vi "svx_Configure (DAQmx).vi"(0 "acquisition task in":T1={"AI device settings"={"AI DAQmx TaskID"="", "response"=[]}, "acquisition type"=enum."Finite", "measurement settings"={"AI sampling frequency"=0.0, "AO sampling frequency"=0.0, "AI block size"=0, "AO block Size"=0, "block duration [ms]"=100.0, "number of AI channels"=0, "device propagation delay [samples]"=0.0, "DUT propagation time [s]"=0.0}, "settling settings"={"settle time"=0.015599999576807022, "settle cycles"=5}, "integration settings"={"integration time"=0.015599999576807022, "integration cycles"=5}, "AO device settings"={"AO DAQmx taskID"="", "excitation"=[]}, "acquisition accounting"={"initial read size [samples]"=0, "read offset [samples]"=0, "read length [samples]"=0, "blocks to settle [samples]"=0, "min delay until transition [samples]"=0}, "frequency range"={"start frequency"=0.0, "stop frequency"=0.0}, "block type"=enum."Initialize", "source settings"={"signal type"=enum."Sine wave", "frequency"=0.0, "total amplitude"=0.0, "frequencies"=[1.0], "relative amplitudes"=[1.0], "offset"=1.0, "total amplitude list"=[1.0], "ramping rate"=0.0}, "chirp settings"={"amplitude"=1.0, "frequency range"={"start (Hz)"=20.0, "stop (Hz)"=20000.0, "frequency spacing"=enum."Logarithmic"}, "sampling info"={"Fs"=50000.0, "chirp duration [s]"=3.0}, "initial states"={"frequency [Hz]"=20.0, "phase [rad]"=0.0, "elapsed time [s]"=0.0}, "frequency slope"=0.0, "maximum harmonic"=3, "prefix len [samples]"={"integer"=0, "fractional"=0.0}}} {"chirp settings"."frequency slope" format="%.2f"; "chirp settings"."prefix len [samples]"."fractional" format="%.2p"; "chirp settings"."initial states"."elapsed time [s]" format="%.2f"; "chirp settings"."initial states"."phase [rad]" format="%.2f"; "chirp settings"."initial states"."frequency [Hz]" format="%.2f"; "chirp settings"."sampling info"."chirp duration [s]" format="%.2f"; "chirp settings"."sampling info"."Fs" format="%.2p"; "chirp settings"."frequency range"."stop (Hz)" format="%.2f"; "chirp settings"."frequency range"."start (Hz)" format="%.2f"; "chirp settings"."amplitude" format="%.2f"; "source settings"."total amplitude" format="%.2f"; "source settings"."relative amplitudes" format="%.2f"; "source settings"."frequencies" format="%.2f"; "source settings"."total amplitude list" format="%.2f"; "source settings"."ramping rate" format="%.4f"; "source settings"."offset" format="%.2f"; "source settings"."frequency" format="%.2f"; "frequency range"."stop frequency" format="%.2f"; "frequency range"."start frequency" format="%.2f"; "AO device settings"."excitation"."AO channel settings"."terminal config" items=["Default"=-1, "Differential"=10106, "Pseudodifferential"=12529]; "AI device settings"."response"."AI channel settings"."DSA channel settings"."IEPE current [mA]" min=0.0 max=20.0 format="%.1f"; "AI device settings"."response"."AI channel settings"."DSA channel settings"."coupling" items=["AC"=10045, "DC"=10050, "GND"=10066]; "AI device settings"."response"."AI channel settings"."min value [V]" format="%.2f"; "AI device settings"."response"."AI channel settings"."terminal config" items=["Default"=-1, "RSE"=10083, "NRSE"=10078, "Differential"=10106, "Pseudodifferential"=12529]; "AI device settings"."response"."AI channel settings"."max value [V]" format="%.2f"; "integration settings"."integration time" format="%.2p"; "settling settings"."settle time" format="%.2p"; "measurement settings"."DUT propagation time [s]" format="%.2f"; "measurement settings"."AO sampling frequency" format="%.2f"; "measurement settings"."AI sampling frequency" format="%.2f"}, 11 "error in (no error)":errorcluster) -> (4 "acquisition task out":T1={"AI device settings"={"AI DAQmx TaskID"="", "response"=[]}, "acquisition type"=enum."Finite", "measurement settings"={"AI sampling frequency"=51200.0, "AO sampling frequency"=51200.0, "AI block size"=0, "AO block Size"=0, "block duration [ms]"=100.0, "number of AI channels"=0, "device propagation delay [samples]"=0.0, "DUT propagation time [s]"=0.0}, "settling settings"={"settle time"=0.015599999576807022, "settle cycles"=5}, "integration settings"={"integration time"=0.015599999576807022, "integration cycles"=5}, "AO device settings"={"AO DAQmx taskID"="", "excitation"=[]}, "acquisition accounting"={"initial read size [samples]"=0, "read offset [samples]"=0, "read length [samples]"=0, "blocks to settle [samples]"=0, "min delay until transition [samples]"=0}, "frequency range"={"start frequency"=0.015599999576807022, "stop frequency"=5.0}, "block type"=enum."Initialize", "source settings"={"signal type"=enum."Sine wave", "frequency"=5.0, "total amplitude"=0.0, "frequencies"=[1.0], "relative amplitudes"=[1.0], "offset"=1.0, "total amplitude list"=[1.0], "ramping rate"=0.0}, "chirp settings"={"amplitude"=1.0, "frequency range"={"start (Hz)"=20.0, "stop (Hz)"=20000.0, "frequency spacing"=enum."Logarithmic"}, "sampling info"={"Fs"=50000.0, "chirp duration [s]"=3.0}, "initial states"={"frequency [Hz]"=20.0, "phase [rad]"=0.0, "elapsed time [s]"=0.0}, "frequency slope"=0.0, "maximum harmonic"=3, "prefix len [samples]"={"integer"=0, "fractional"=0.0}}} {"chirp settings"."frequency slope" format="%.2f"; "chirp settings"."prefix len [samples]"."fractional" format="%.2p"; "chirp settings"."initial states"."elapsed time [s]" format="%.2f"; "chirp settings"."initial states"."phase [rad]" format="%.2f"; "chirp settings"."initial states"."frequency [Hz]" format="%.2f"; "chirp settings"."sampling info"."chirp duration [s]" format="%.2f"; "chirp settings"."sampling info"."Fs" format="%.2p"; "chirp settings"."frequency range"."stop (Hz)" format="%.2f"; "chirp settings"."frequency range"."start (Hz)" format="%.2f"; "chirp settings"."amplitude" format="%.2f"; "source settings"."total amplitude" format="%.2f"; "source settings"."relative amplitudes" format="%.2f"; "source settings"."frequencies" format="%.2f"; "source settings"."total amplitude list" format="%.2f"; "source settings"."ramping rate" format="%.4f"; "source settings"."offset" format="%.2f"; "source settings"."frequency" format="%.2f"; "frequency range"."stop frequency" format="%.2f"; "frequency range"."start frequency" format="%.2f"; "AO device settings"."excitation"."AO channel settings"."terminal config" items=["Default"=-1, "Differential"=10106, "Pseudodifferential"=12529]; "AI device settings"."response"."AI channel settings"."DSA channel settings"."IEPE current [mA]" min=0.0 max=20.0 format="%.1f"; "AI device settings"."response"."AI channel settings"."DSA channel settings"."coupling" items=["AC"=10045, "DC"=10050, "GND"=10066]; "AI device settings"."response"."AI channel settings"."min value [V]" format="%.2f"; "AI device settings"."response"."AI channel settings"."terminal config" items=["Default"=-1, "RSE"=10083, "NRSE"=10078, "Differential"=10106, "Pseudodifferential"=12529]; "AI device settings"."response"."AI channel settings"."max value [V]" format="%.2f"; "integration settings"."integration time" format="%.2p"; "settling settings"."settle time" format="%.2p"; "measurement settings"."DUT propagation time [s]" format="%.2f"; "measurement settings"."AO sampling frequency" format="%.2f"; "measurement settings"."AI sampling frequency" format="%.2f"}, 6 "actual scan rate":dbl format="%.2f", 15 "error out":errorcluster)   [LabVIEW 2017]
uses:
  <vilib>/addons/Sound and Vibration/Example Support/Audio/DAQmx/svx_Acquisition Task (DAQmx).ctl
  <vilib>/addons/_NISVFA/_Shared subVIs/Controls/svc_Channel Settings.ctl
  <vilib>/addons/_NISVFA/_Shared subVIs/Controls/svc_DSA Channel Settings.ctl
  <vilib>/addons/_NISVFA/_Generation/subVIs/sv_Chirp Settings.ctl
  <vilib>/DAQmx/configure/trigger.llb/DAQmx Start Trigger (Digital Edge).vi
  <vilib>/DAQmx/configure/timing.llb/DAQmx Timing (Sample Clock).vi
  <vilib>/DAQmx/create/channels.llb/DAQmx Create Channel (AO-Voltage-Basic).vi
  <vilib>/DAQmx/create/channels.llb/DAQmx Create Channel (AI-Voltage-Basic).vi
  <resource>/objmgr/daqmx.rc
  <vilib>/addons/_NISVFA/_Generation/SoundVib_Generation.lvlib
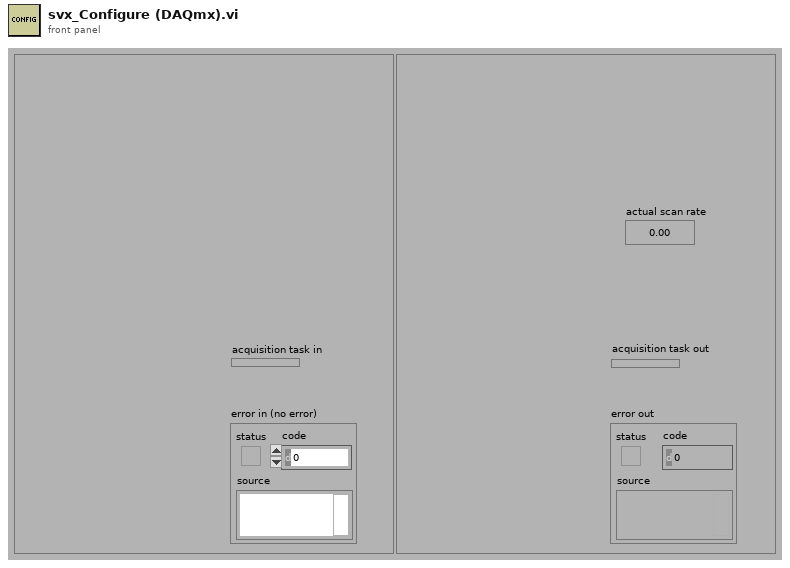
[diagram p1: front panel]
types:
  T1 = typedef "svx_Acquisition Task (DAQmx).ctl" = cluster{"AI device settings":cluster{"AI DAQmx TaskID":refnum<k21>, "response":cluster{"AI physical channel":tag, "AI channel settings":T2}[]}, "acquisition type":enum16{"Finite", "Averaged", "Settled", "Amplitude Sweep", "Stepped Frequency Sweep", "Continuous Frequency Sweep"}, "measurement settings":cluster{"AI sampling frequency":dbl, "AO sampling frequency":dbl, "AI block size":i32, "AO block Size":i32, "block duration [ms]":dbl, "number of AI channels":i32, "device propagation delay [samples]":dbl, "DUT propagation time [s]":dbl}, "settling settings":cluster{"settle time":dbl, "settle cycles":i32}, "integration settings":cluster{"integration time":dbl, "integration cycles":i32}, "AO device settings":cluster{"AO DAQmx taskID":refnum<k21>, "excitation":cluster{"AO physical channel":tag, "AO channel settings":cluster{"maximum value (10 V)":dbl, "minimum value (10 V)":dbl, "terminal config":i32}}[]}, "acquisition accounting":cluster{"initial read size [samples]":i32, "read offset [samples]":i32, "read length [samples]":i32, "blocks to settle [samples]":i32, "min delay until transition [samples]":i32}, "frequency range":cluster{"start frequency":dbl, "stop frequency":dbl}, "block type":enum16{"Initialize", "Settle", "Integrate"}, "source settings":cluster{"signal type":enum16{"Sine wave", "Dual tone (IMD)", "Multitone", "Chirp", "Frequency flat chirp", "Uniform white noise", "Gaussian white noise", "Pink noise", "PRN", "Continuous swept-sine"}, "frequency":dbl, "total amplitude":dbl, "frequencies":dbl[], "relative amplitudes":dbl[], "offset":dbl, "total amplitude list":dbl[], "ramping rate":dbl}, "chirp settings":T4}
  T2 = typedef "svc_Channel Settings.ctl" = cluster{"max value [V]":dbl, "min value [V]":dbl, "terminal config":i32, "DSA channel settings":T3}
  T3 = typedef "svc_DSA Channel Settings.ctl" = cluster{"coupling":i32, "enable IEPE excitation":bool, "IEPE current [mA]":dbl}
  T4 = typedef "SoundVib_Generation.lvlib/sv_Chirp Settings.ctl" = cluster{"amplitude":dbl, "frequency range":cluster{"start (Hz)":dbl, "stop (Hz)":dbl, "frequency spacing":enum16{"Linear", "Logarithmic"}}, "sampling info":cluster{"Fs":dbl, "chirp duration [s]":dbl}, "initial states":cluster{"frequency [Hz]":dbl, "phase [rad]":dbl, "elapsed time [s]":dbl}, "frequency slope":dbl, "maximum harmonic":i32, "prefix len [samples]":cluster{"integer":u32, "fractional":dbl}}
  T5 = enum16{"Finite", "Averaged", "Settled", "Amplitude Sweep", "Stepped Frequency Sweep", "Continuous Frequency Sweep"}
  T6 = cluster{"AO physical channel":tag, "AO channel settings":cluster{"maximum value (10 V)":dbl, "minimum value (10 V)":dbl, "terminal config":i32}}[]
  T7 = cluster{"AI physical channel":tag, "AI channel settings":T2}[]
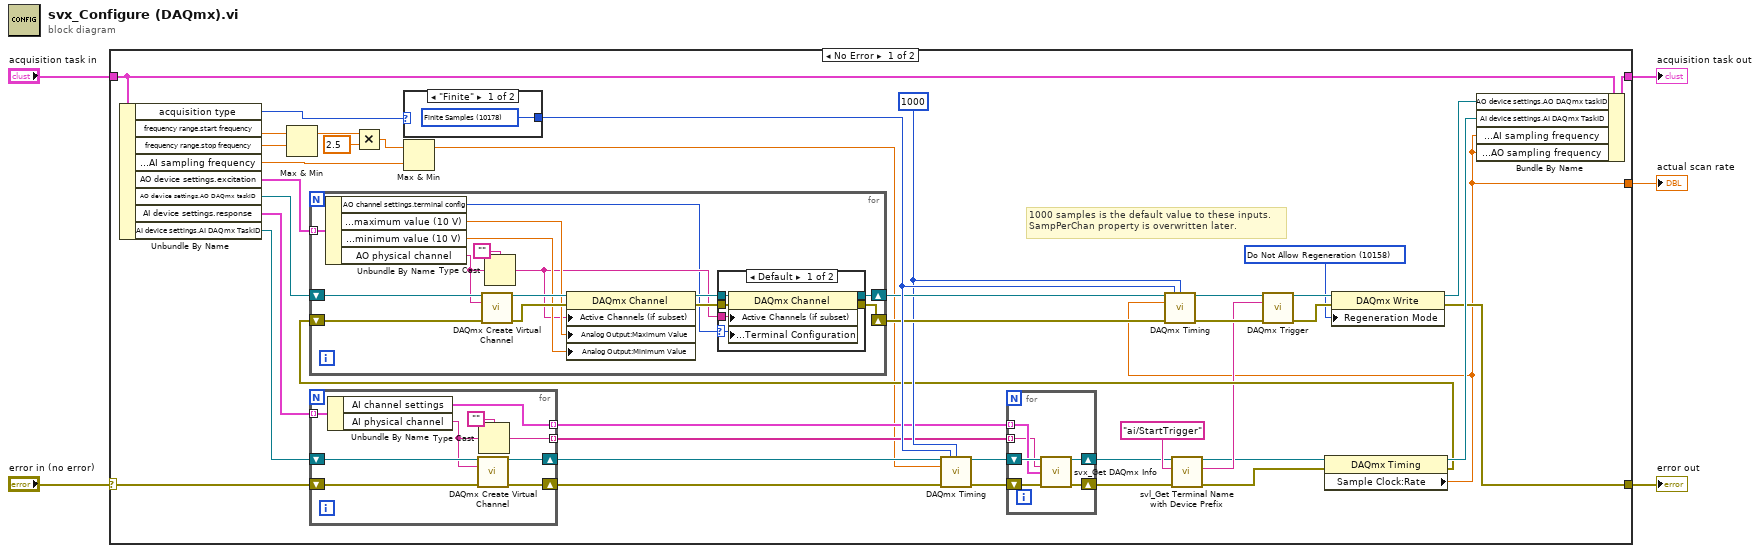
[diagram p0: block diagram]
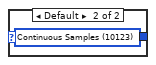
[diagram p3: hidden frame]
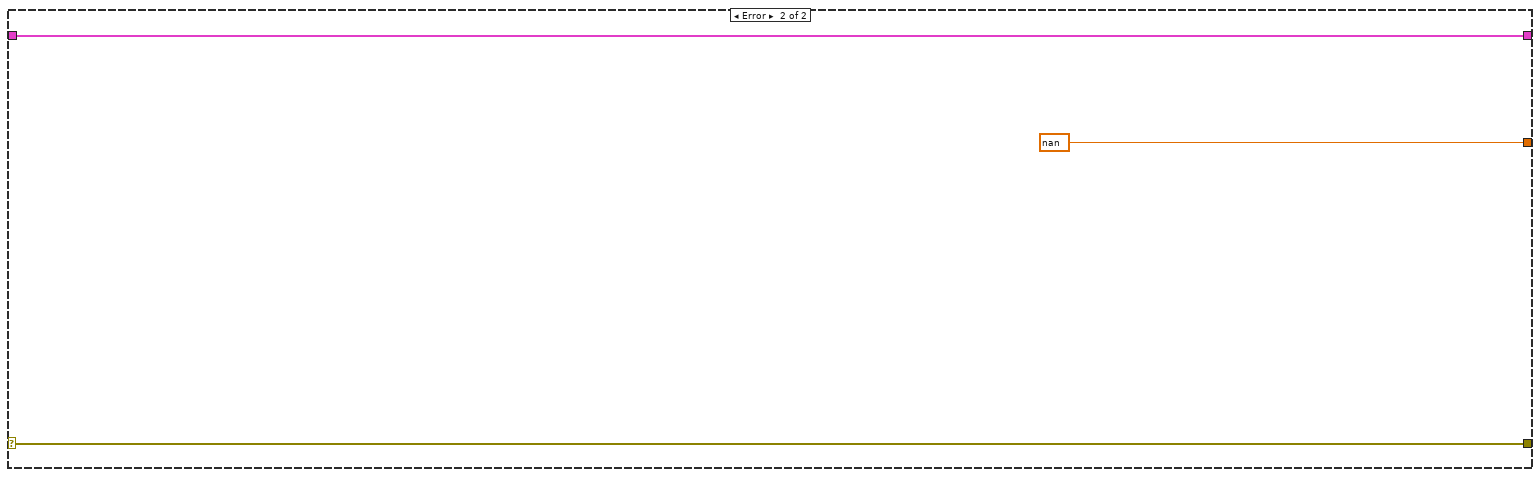
[diagram p4: hidden frame]
diagram:
  n1 = case shown="No Error" "error in (no error)" {
    selector: "error in (no error)" -> [w37 w87]
    tunnel: "acquisition task in" -> [w46 w89]
    tunnel: [w21 w87] -> w4
    tunnel: [w13 nan ("SampClk.Rate")] -> w3
    tunnel: [w40 w89] -> w2
    frame No Error {
      w26 = 1000 ("samples per channel")
      w41 = 10158 items=["Allow Regeneration"=10097, "Do Not Allow Regeneration"=10158] ("RegenMode")
      # "1000 samples is the default value to these inputs.\nSampPerChan property is overwritten later."
      n2 = Unbundle By Name(w46) -> ("acquisition type"=w39:T5, "frequency range.start frequency"=w12:dbl, "frequency range.stop frequency"=w11:dbl, "measurement settings.AI sampling frequency"=w7:dbl, "AO device settings.excitation"=w33:T6, "AO device settings.AO DAQmx taskID"=w36:refnum<k21>, "AI device settings.response"=w32:T7, "AI device settings.AI DAQmx TaskID"=w31:refnum<k21>)
      n3 = Max & Min(x=w12, y=w11) -> (max(x,y)=w9:dbl)  [unwired: 1 out]
      n4 = for {
        shift-right: [w78] -> w27
        shift-left: w37 -> [w84]
        shift-right: [w79] -> w28
        shift-left: w31 -> [w83]
        tunnel: w32 -> [w82] mode=indexing
        tunnel: [w77] -> w23 mode=indexing
        tunnel: [w76] -> w22 mode=indexing
        n5 = Unbundle By Name(w82) -> ("AI channel settings"=w77:T2, "AI physical channel"=w80:tag)
        n6 = call-poly <vilib>:"DAQmx Create Virtual Channel.vi"("task in"=w83, "physical channels"=w80, "error in"=w84) -> ("task out"=w79:refnum<k21>, "error out"=w78:errorcluster)  [unwired: 11 in]
        n7 = Type Cast(type="" ("active channels"), x=w80) -> (*(type *) &x=w76:string)
      }
      n8 = Multiply(x=w9, y=2.5) -> (x*y=w8:dbl)
      n9 = case shown="\"Finite\"" w39 {
        tunnel: [w85 w86] -> w38
        frame "Finite" {
          w85 = 10178 items=["Finite Samples"=10178, "Continuous Samples"=10123] ("sample mode")
        }
        frame Default {
          w86 = 10123 items=["Finite Samples"=10178, "Continuous Samples"=10123] ("sample mode")
        }
      }
      n10 = Max & Min(x=w8, y=w7) -> (max(x,y)=w6:dbl)  [unwired: 1 out]
      n11 = call-poly <vilib>:"DAQmx Timing.vi"("task/channels in"=w28, "sample mode"=w38, "samples per channel"=w26, "rate"=w6, "error in"=w27) -> ("task out"=w25:refnum<k21>, "error out"=w24:errorcluster)  [unwired: 9 in]
      n12 = for {
        shift-right: [w51] -> w19
        shift-left: w25 -> [w52]
        shift-right: [w49] -> w18
        shift-left: w24 -> [w50]
        tunnel: w23 -> [w48] mode=indexing
        tunnel: w22 -> [w47] mode=indexing
        n13 = call <vilib>:"svx_Get DAQmx Info.vi"("task in"=w52, "active channels"=w47, "AI channel settings"=w48, "error in (no error)"=w50) -> ("task out"=w51:refnum<k21>, "error out"=w49:errorcluster)  [unwired: 10 in]
      }
      n14 = call <vilib>:"svl_Get Terminal Name with Device Prefix.vi"("error in (no error)"=w18, "local terminal name"="ai/StartTrigger", "task/channels in"=w19) -> ("error out"=w14:errorcluster, "terminal name with device prefix"=w16:tag, "task out"=w15:refnum<k21>)  [unwired: 6 in]
      n15 = property class="DAQmx Timing"(reference=w15, error in=w14) -> (reference out=w30:refnum<k21>, error out=w17:errorcluster, "Sample Clock:Rate"=w13:dbl)
      n16 = for {
        shift-right: [w54] -> w34
        shift-left: w17 -> [w65]
        shift-right: [w56] -> w35
        shift-left: w36 -> [w66]
        tunnel: w33 -> [w67] mode=indexing
        n17 = Unbundle By Name(w67) -> ("AO channel settings.terminal config"=w53:i32, "AO channel settings.maximum value (10 V)"=w60:dbl, "AO channel settings.minimum value (10 V)"=w59:dbl, "AO physical channel"=w61:tag)
        n18 = call-poly <vilib>:"DAQmx Create Virtual Channel.vi"("task in"=w66, "physical channels"=w61, "error in"=w65) -> ("task out"=w64:refnum<k21>, "error out"=w63:errorcluster)  [unwired: 11 in]
        n19 = Type Cast(type="" ("active channels"), x=w61) -> (*(type *) &x=w55:string)
        n20 = property class="DAQmx Channel"(reference=w64, error in=w63, "Active Channels (if subset)"=w55, "Analog Output:Maximum Value"=w60, "Analog Output:Minimum Value"=w59) -> (reference out=w58:refnum<k21>, error out=w57:errorcluster)
        n21 = case shown="Default" w53 {
          selector: w53 -> [w68 _]
          tunnel: w58 -> [w73 w75]
          tunnel: w57 -> [w72 w74]
          tunnel: [w71 w75] -> w56
          tunnel: w55 -> [w70 _]
          tunnel: [w69 w74] -> w54
          frame Default {
            n22 = property class="DAQmx Channel"(reference=w73, error in=w72, "Active Channels (if subset)"=w70, "Analog Output:General Properties:Output Configuration:Terminal Configuration"=w68) -> (reference out=w71:refnum<k21>, error out=w69:errorcluster)
          }
          frame -1 {
          }
        }
      }
      n23 = call-poly <vilib>:"DAQmx Timing.vi"("task/channels in"=w35, "sample mode"=w38, "samples per channel"=w26, "rate"=w13, "error in"=w34) -> ("task out"=w45:refnum<k21>, "error out"=w44:errorcluster)  [unwired: 9 in]
      n24 = call-poly <vilib>:"DAQmx Trigger.vi"("task/channels in"=w45, "source"=w16, "error in"=w44) -> ("task out"=w43:refnum<k21>, "error out"=w42:errorcluster)  [unwired: 11 in]
      n25 = property class="DAQmx Write"(reference=w43, error in=w42, "Regeneration Mode"=w41) -> (reference out=w29:refnum<k21>, error out=w21:errorcluster)
      n26 = Bundle By Name(cluster=w46, "AO device settings.AO DAQmx taskID"=w29, "AI device settings.AI DAQmx TaskID"=w30, "measurement settings.AI sampling frequency"=w13, "measurement settings.AO sampling frequency"=w13) -> (w40:T1)
    }
    frame Error {
    }
  }
  "actual scan rate" <- w3
  "error out" <- w4
  "acquisition task out" <- w2
